vi "Determine Warnings 3-9.vi"() -> ()   [LabVIEW 2014]
panel:
  in  "Max Wind Speed":dbl
  in  "Current Wind Speed":dbl
  out "Warning?":bool
  out "Warning Text":string
  in  "Min Temp":dbl
  in  "Max Temp":dbl
  in  "Current Temp":dbl
  # "If you have a min temp that is greater than your max temp then the warning text will be \ndetermined by the the Current Temps value"
  # "18."
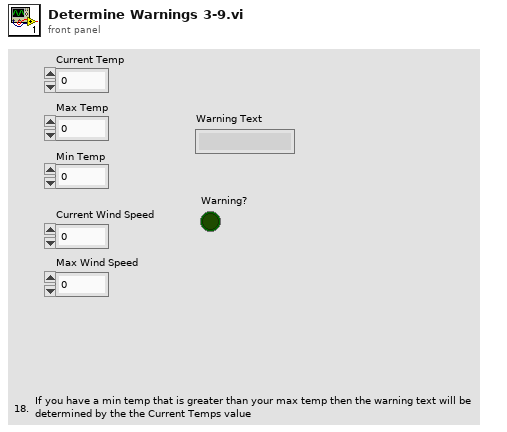
[diagram p1: front panel]
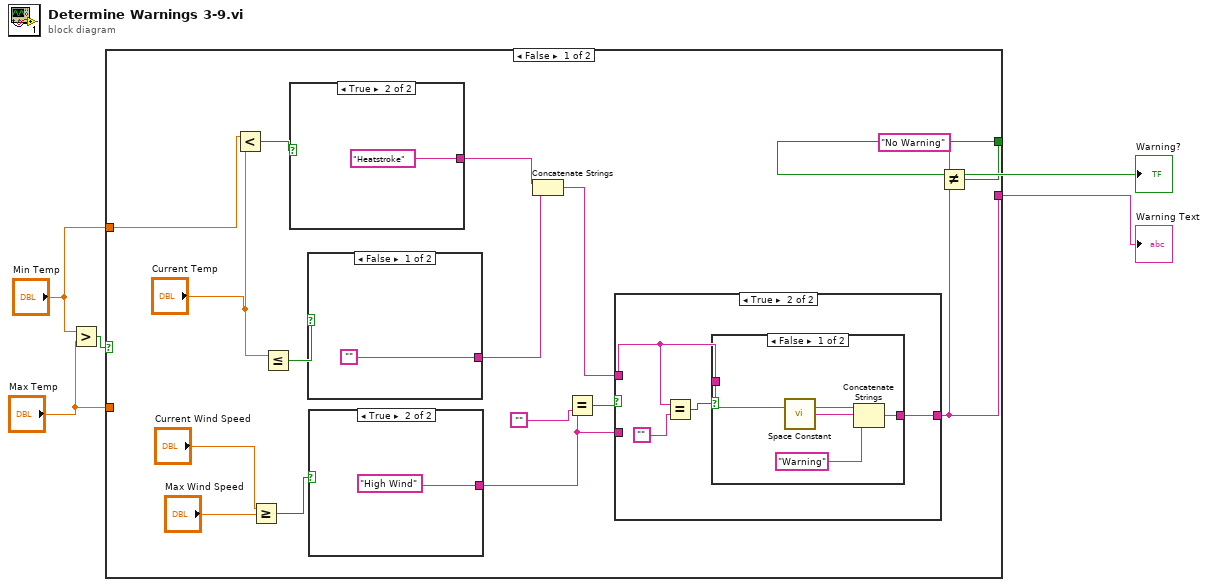
[diagram p0: block diagram]
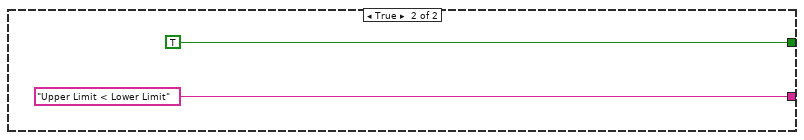
[diagram p7: hidden frame]
diagram:
  n1 = Greater?(x="Min Temp", y="Max Temp") -> (0:w1:bool)
  n2 = case shown="False" w1 {
    tunnel: [w13 TRUE] -> w5
    tunnel: [w11 "Upper Limit < Lower Limit"] -> w4
    tunnel: "Min Temp" -> [w21 _]
    tunnel: "Max Temp" -> [_ _]
    frame False {
      n3 = Less?(x=w21, y="Current Temp") -> (x < y?=w7:bool)
      n4 = Greater Or Equal?(x="Current Wind Speed", y="Max Wind Speed") -> (x >= y?=w17:bool)
      n5 = Less Or Equal?(x="Current Temp") -> (x <= y?=w6:bool)  [unwired: 1 in]
      n6 = case shown="True" w7 {
        tunnel: [_ "Heatstroke"] -> w16
        frame False {
        }
        frame True {
        }
      }
      n7 = case shown="False" w6 {
        tunnel: ["" _] -> w15
        frame False {
        }
        frame True {
        }
      }
      n8 = case shown="True" w17 {
        tunnel: [_ "High Wind"] -> w8
        frame False {
        }
        frame True {
        }
      }
      n9 = Concatenate Strings(w16, w15) -> (w14:string)
      n10 = Equal?(x=w8, y="") -> (x = y?=w9:bool)
      n11 = case shown="True" w9 {
        tunnel: w14 -> [_ w22]
        tunnel: [_ w24] -> w11
        tunnel: w8 -> [_ _]
        frame False {
        }
        frame True {
          n12 = Equal?(x=w22, y="") -> (x = y?=w25:bool)
          n13 = case shown="False" w25 {
            tunnel: w22 -> [w29 _]
            tunnel: [w26 _] -> w24
            frame False {
              n14 = call <vilib>:"Space Constant.vi"() -> ("String"=w28:string)
              n15 = Concatenate Strings(w29, w28, "Warning") -> (w26:string)
            }
            frame True {
            }
          }
        }
      }
      n16 = Not Equal?(x="No Warning", y=w11) -> (x != y?=w13:bool)
    }
    frame True {
    }
  }
  "Warning Text" <- w4
  "Warning?" <- w5
